vi "radyProwadzacego.vi"() -> ()   [LabVIEW 2018]
uses:
  <vilib>/Utility/miscctls.llb/LVDateTimeRec.ctl
panel:
  out "date/time string":string
  in  "Array":string[][](array[string])
  out "time stamp":timestamp
  in  "date time rec":T1
  in  "date format (0)":enum16{"short", "long", "abbreviated"}(ring)
  out "current time":timestamp
  out "time string":string
  out "date string":string
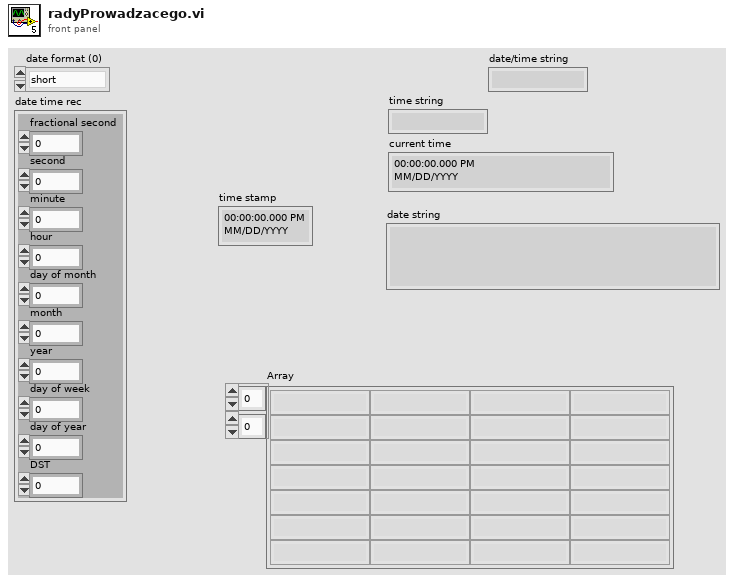
[diagram p1: front panel]
types:
  T1 = typedef "LVDateTimeRec.ctl" = cluster{"fractional second":dbl, "second":i32, "minute":i32, "hour":i32, "day of month":i32, "month":i32, "year":i32, "day of week":i32, "day of year":i32, "DST":i32}
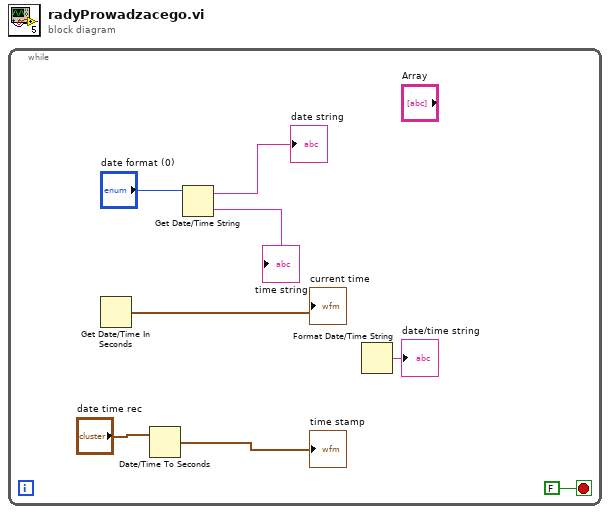
[diagram p0: block diagram]
diagram:
  n1 = while {
    stop <- FALSE stop-if-true
    n2 = Get Date/Time In Seconds() -> (seconds since 1Jan1904=→"current time":timestamp)
    n3 = Date/Time To Seconds(2:"date time rec") -> (0:→"time stamp":timestamp)  [unwired: 1 in]
    n4 = Get Date/Time String(date format (0)="date format (0)") -> (date string=→"date string":string, time string=→"time string":string)  [unwired: 2 in]
    n5 = Format Date/Time String() -> (date/time string=→"date/time string":string)  [unwired: 3 in]
  }
